vi "RW_RobotMacros.vi"(7 "Action":enum16{"read", "write"}(ring), 10 "Macros":T1[](array[typedef]) {"Sequence"."Axes 2"."Switch" format="%#_4g"; "Sequence"."Axes 2"."Axis 2" format="%#_4g"; "Sequence"."Axes 2"."Axis 1" format="%#_4g"; "Sequence"."Axes 2"."Axis 0" format="%#_4g"; "Sequence"."Axes 1"."Axis 6" format="%#_4g"; "Sequence"."Axes 1"."Axis 5" format="%#_4g"; "Sequence"."Axes 1"."Axis 4" format="%#_4g"; "Sequence"."Axes 1"."Axis 3" format="%#_4g"; "Sequence"."Axes 1"."Axis 2" format="%#_4g"; "Sequence"."Axes 1"."Axis 1" format="%#_4g"}, 11 "File Path":path=path "c:/RobotMacros.cfg") -> (0 "error out":errorcluster, 2 "Macros out":T1[](array[typedef]) {"Sequence"."Axes 2"."Switch" format="%#_4g"; "Sequence"."Axes 2"."Axis 2" format="%#_4g"; "Sequence"."Axes 2"."Axis 1" format="%#_4g"; "Sequence"."Axes 2"."Axis 0" format="%#_4g"; "Sequence"."Axes 1"."Axis 6" format="%#_4g"; "Sequence"."Axes 1"."Axis 5" format="%#_4g"; "Sequence"."Axes 1"."Axis 4" format="%#_4g"; "Sequence"."Axes 1"."Axis 3" format="%#_4g"; "Sequence"."Axes 1"."Axis 2" format="%#_4g"; "Sequence"."Axes 1"."Axis 1" format="%#_4g"})   [LabVIEW 2017]
uses:
  Ctrl Refs/Macros.ctl
  Ctrl Refs/JoyStick1.ctl
  Ctrl Refs/JoyStick1(Analog).ctl
  Ctrl Refs/JoyStick2.ctl
  Ctrl Refs/JoyStick2(Analog).ctl
panel:
  in  "Tab Control":enum32{"Inputs", "Outputs"}(tab)
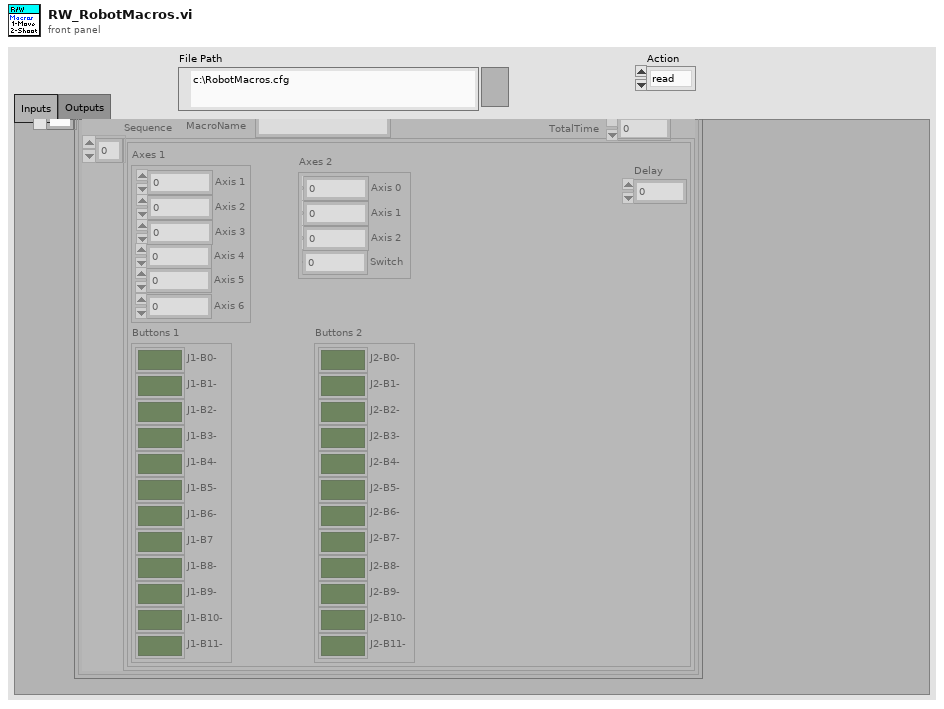
[diagram p1: front panel]
types:
  T1 = typedef "Macros.ctl" = cluster{"MacroName":string, "Sequence":cluster{"Buttons 1":T2, "Axes 1":T3, "Buttons 2":T4, "Axes 2":T5, "Delay":u32}[], "TotalTime":u32}
  T2 = typedef "JoyStick1.ctl" = cluster{"J1-B0-":bool, "J1-B1-":bool, "J1-B2-":bool, "J1-B3- ":bool, "J1-B4-":bool, "J1-B5-":bool, "J1-B6-":bool, "J1-B7":bool, "J1-B8-":bool, "J1-B9-":bool, "J1-B10-":bool, "J1-B11-":bool}
  T3 = typedef "JoyStick1(Analog).ctl" = cluster{"Axis 1":dbl, "Axis 2":dbl, "Axis 3":dbl, "Axis 4":dbl, "Axis 5":dbl, "Axis 6":dbl}
  T4 = typedef "JoyStick2.ctl" = cluster{"J2-B0-":bool, "J2-B1-":bool, "J2-B2-":bool, "J2-B3-":bool, "J2-B4-":bool, "J2-B5-":bool, "J2-B6-":bool, "J2-B7-":bool, "J2-B8-":bool, "J2-B9-":bool, "J2-B10-\n":bool, "J2-B11-":bool}
  T5 = typedef "JoyStick2(Analog).ctl" = cluster{"Axis 0":dbl, "Axis 1":dbl, "Axis 2":dbl, "Switch":dbl}
  T6 = enum16{"open", "replace", "create", "open or create", "replace or create", "replace or create with confirmation"}
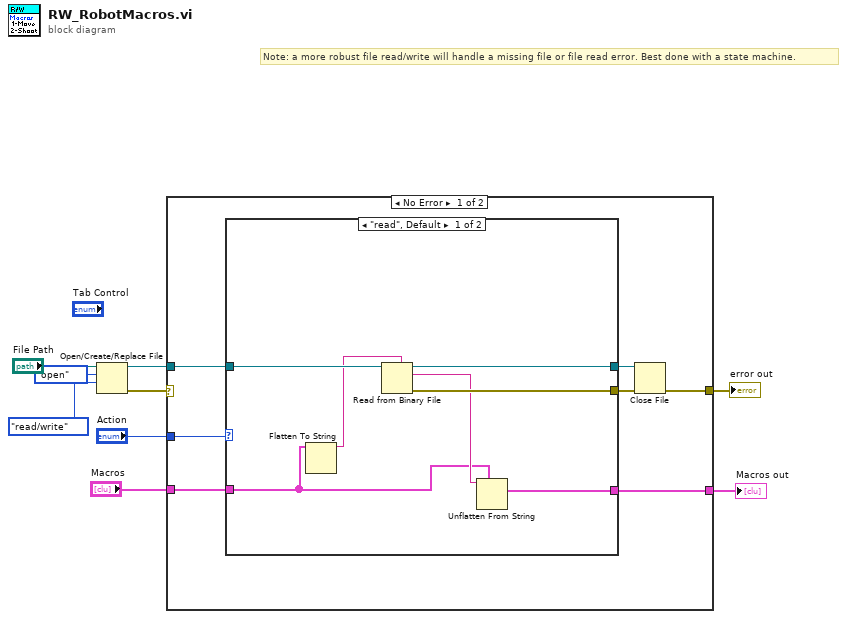
[diagram p0: block diagram]
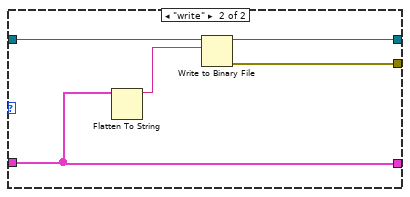
[diagram p2: hidden frame]
diagram:
  # "Note: a more robust file read/write will handle a missing file or file read error. Best done with a state machine."
  n1 = Open/Create/Replace File(file path (use dialog)="File Path", operation (0:open)=T6."open", access (0:read/write)=enum16{"read/write", "read-only", "write-only"}."read/write") -> (refnum out=w7:refnum<file>, error out=w8:errorcluster)  [unwired: 3 in, 1 out]
  n2 = case shown="No Error" w8 {
    selector: w8 -> [_ w30]
    tunnel: w7 -> [w15 _]
    tunnel: "Action" -> [w16 _]
    tunnel: "Macros" -> [w14 w29]
    tunnel: [w11 w30] -> w4
    tunnel: [w10 w29] -> w3
    frame No Error {
      n3 = case shown="\"read\", Default" w16 {
        tunnel: w15 -> [w23 w28]
        tunnel: w14 -> [w17 w24]
        tunnel: [w19 w26] -> w13
        tunnel: [w22 w25] -> w12
        tunnel: [w20 w24] -> w10
        frame "read", Default {
          n4 = Flatten To String(anything=w17) -> (data string=w18:string)  [unwired: 3 in, 2 out]
          n5 = Read from Binary File(5:w18, 11:w23) -> (0:w22:errorcluster, 2:w21:string, 3:w19:refnum<file>)  [unwired: 4 in, 1 out]
          n6 = Unflatten From String(type=w17, binary string=w21) -> (value=w20:T1[])  [unwired: 3 in, 2 out]
        }
        frame "write" {
          n7 = Flatten To String(anything=w24) -> (data string=w27:string)  [unwired: 3 in, 2 out]
          n8 = Write to Binary File(file (use dialog)=w28, data=w27) -> (refnum out=w26:refnum<file>, error out=w25:errorcluster)  [unwired: 4 in, 1 out]
        }
      }
      n9 = Close File(refnum=w13, error in=w12) -> (error out=w11:errorcluster)  [unwired: 1 out]
    }
    frame Error {
    }
  }
  "error out" <- w4
  "Macros out" <- w3
